vi "Setup UI.vi"(8 "error in (no error)":errorcluster, 10 "Set UI to input?":bool, 11 "File IO in":refnum<class "File IO.lvclass">) -> (0 "error out":errorcluster, 3 "File IO out":refnum<class "File IO.lvclass">)   [LabVIEW 2009, in "File IO.lvclass"]
uses:
  File IO.lvclass
  File IO.lvclass/File IO.ctl
panel:
  in  "Light Source":string
  in  "Comments":string
  in  "File Path":path
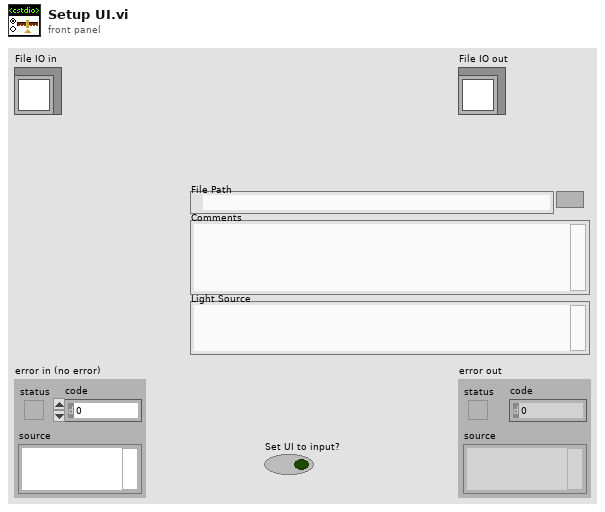
[diagram p1: front panel]
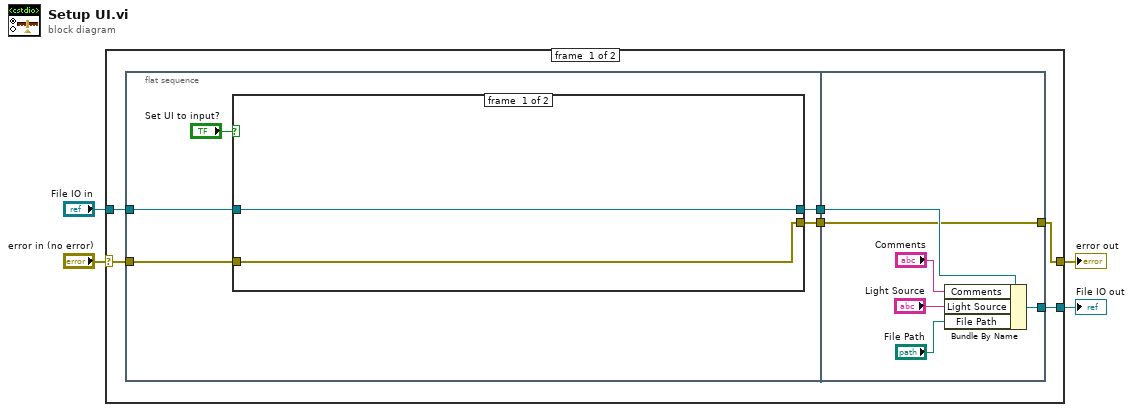
[diagram p0: block diagram]
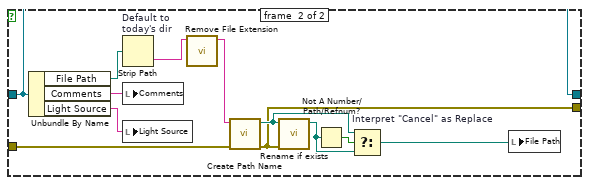
[diagram p2: hidden frame]
diagram:
  n1 = case shown="No Error" "error in (no error)" {
    selector: "error in (no error)" -> [w7 w37]
    tunnel: [w5 w37] -> w3
    tunnel: [w9 w36] -> w1
    tunnel: "File IO in" -> [w10 w36]
    frame #0 {
      n2 = flat-sequence {
        tunnel: w10 -> [w14]
        tunnel: [w13] -> w8
        tunnel: w7 -> [w12]
        tunnel: [w11] -> w6
        tunnel: [w35] -> w9
        tunnel: w8 -> [w32]
        tunnel: w6 -> [w30]
        tunnel: [w30] -> w5
        frame #0 {
          n3 = case shown="True" "Set UI to input?" {
            tunnel: w14 -> [w16 w29]
            tunnel: [w16 w29] -> w13
            tunnel: w12 -> [w17 w25]
            tunnel: [w17 w18] -> w11
            frame #0 {
            }
            frame #1 {
              n4 = Unbundle By Name(w29) -> ("File Path"=w26:path, "Comments"=w28:string, "Light Source"=w27:string)
              n5 = Strip Path "Default to\ntoday's dir"(path=w26) -> (name=w24:string)  [unwired: 1 out]
              n6 = local write "Comments"(w28) -> ()
              n7 = local write "Light Source"(w27) -> ()
              n8 = call "Remove File Extension.vi"("filename"=w24) -> ("adjustedfilename"=w23:string)  [unwired: 6 out]
              n9 = call "Create Path Name.vi"("error in"=w25, "filename"=w23) -> ("error out"=w18:errorcluster, "path"=w20:path)  [unwired: 4 out]
              n10 = call "Rename if exists.vi"("error in"=w18, "File Path"=w20) -> ("New path"=w22:path)  [unwired: 1 in, 8 out]
              n11 = Not A Number/Path/Refnum?(number/path/refnum=w22) -> (NaN/Path/Refnum?=w21:bool)
              n12 = Select "Interpret \"Cancel\" as Replace"(t=w20, s=w21, f=w22) -> (s? t:f=w19:path)
              n13 = local write "File Path"(w19) -> ()
            }
          }
        }
        frame #1 {
          n14 = Bundle By Name(cluster=w32, "Comments"="Comments", "Light Source"="Light Source", "File Path"="File Path") -> (w35:refnum<class "File IO.lvclass">)
        }
      }
    }
    frame #1 {
    }
  }
  "error out" <- w3
  "File IO out" <- w1
